vi "Indicator Sub.vi"() -> (1 "Robot Lift Lower":bool, 2 "Robot Lift Upper":bool, 3 "Cube Lift":bool)   [LabVIEW 2017]
uses:
  <vilib>/Rock Robotics/Network Tables/NT Read Boolean.vi
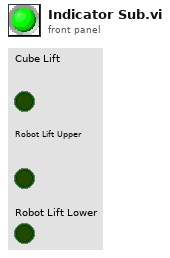
[diagram p1: front panel]
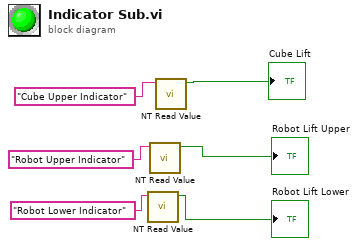
[diagram p0: block diagram]
diagram:
  n1 = call-poly <vilib>:"NT Read Value.vi"("Name"="Robot Lower Indicator") -> ("Boolean"=→"Robot Lift Lower":bool)  [unwired: 9 in, 1 out]
  n2 = call-poly <vilib>:"NT Read Value.vi"("Name"="Robot Upper Indicator") -> ("Boolean"=→"Robot Lift Upper":bool)  [unwired: 9 in, 1 out]
  n3 = call-poly <vilib>:"NT Read Value.vi"("Name"="Cube Upper Indicator") -> ("Boolean"=→"Cube Lift":bool)  [unwired: 9 in, 1 out]
